vi "SetAllPath.vi"(0 "拆分的路径":path, 1 "布尔":bool, 5 "error in (no error)":errorcluster caption="错误输入（无错误）") -> (14 "MainPath":path, 15 "ModelInformation":path, 16 "ConfigPath":path, 17 "LogPath":path, 19 "error out":errorcluster caption="错误输出")   [LabVIEW 2018]
uses:
  Global.vi
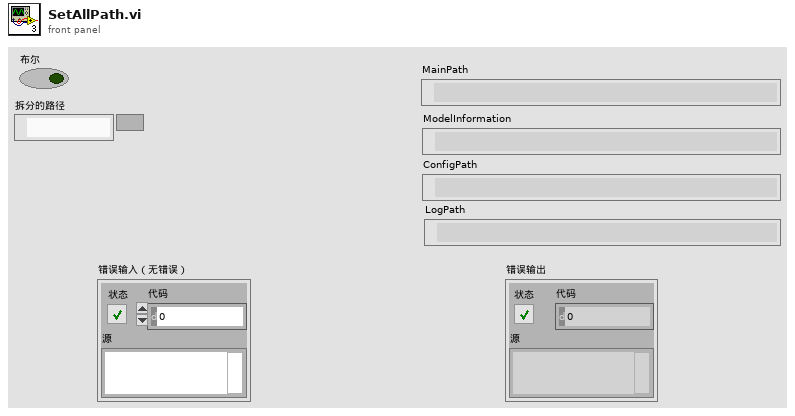
[diagram p1: front panel]
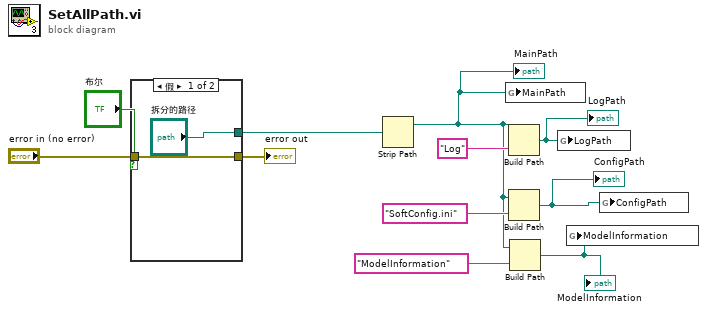
[diagram p0: block diagram]
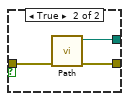
[diagram p2: hidden frame]
diagram:
  n1 = case shown="假" "布尔" {
    tunnel: ["拆分的路径" w16] -> w10
    tunnel: "error in (no error)" -> [w12 w15]
    tunnel: [w12 w14] -> w8
    frame False {
    }
    frame True {
      n2 = call "Path.vi"("error in (no error)"=w15) -> ("error out"=w14:errorcluster, "拆分的路径"=w16:path)  [unwired: 9 in]
    }
  }
  "error out" <- w8
  n3 = Strip Path(path=w10) -> (stripped path=w3:path)  [unwired: 1 out]
  "MainPath" <- w3
  n4 = global write "Global.vi" "MainPath"(w3) -> ()
  n5 = Build Path(base path=w3, name or relative path="Log" ("名称或相对路径")) -> (appended path=w2:path)
  "LogPath" <- w2
  n6 = Build Path(base path=w3, name or relative path="SoftConfig.ini" ("名称或相对路径")) -> (appended path=w4:path)
  "ConfigPath" <- w4
  n7 = Build Path(base path=w3, name or relative path="ModelInformation" ("名称或相对路径")) -> (appended path=w6:path)
  "ModelInformation" <- w6
  n8 = global write "Global.vi" "LogPath"(w2) -> ()
  n9 = global write "Global.vi" "ModelInformation"(w6) -> ()
  n10 = global write "Global.vi" "ConfigPath"(w4) -> ()
